vi "CRYHarmonics list to array.vi"(10 "Checkoffs":bool[](array[boolean]), 11 "Harmonic list items":string[](array[string])) -> (2 "List items checked":string[](array[string]), 3 "Harmonics array out":dbl[](array[numeric]) format="%.2f")   [LabVIEW 2013]
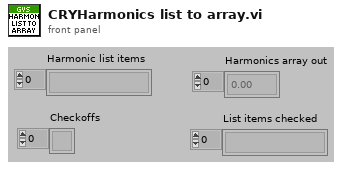
[diagram p1: front panel]
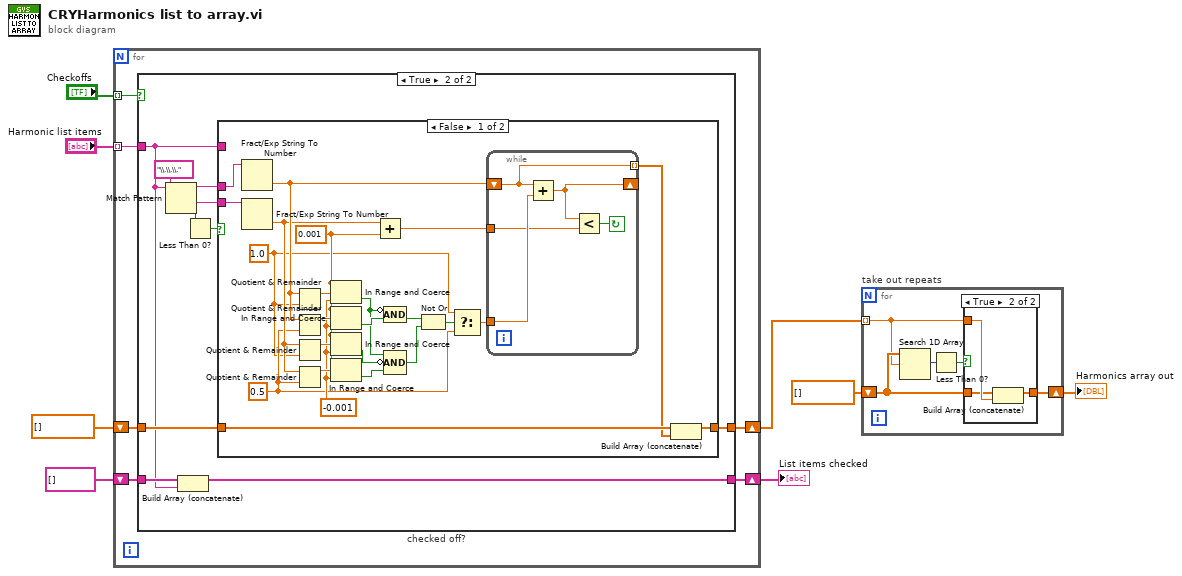
[diagram p0: block diagram]
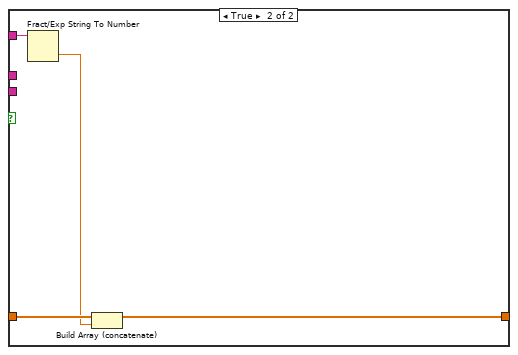
[diagram p4: hidden frame]
diagram:
  n1 = for {
    tunnel: "Checkoffs" -> [w14] mode=indexing
    shift-right: [w11] -> w3
    shift-left: dbl[] [] ("Harmonics array out") -> [w12]
    tunnel: "Harmonic list items" -> [w13] mode=indexing
    shift-right: [w9] -> w4
    shift-left: string[] [] ("Harmonic list items") -> [w10]
    n2 = case "checked off?" shown="True" w14 {
      tunnel: w13 -> [_ w18]
      tunnel: [w16 w20] -> w11
      tunnel: w12 -> [w16 w21]
      tunnel: w10 -> [w15 w19]
      tunnel: [w15 w17] -> w9
      frame False {
      }
      frame True {
        n3 = Match Pattern(string=w18, regular expression="\\.\\.\\.") -> (before substring=w23:string, after substring=w22:string, offset past match=w25:i32)  [unwired: 2 out]
        n4 = Build Array (concatenate)(w19, w18) -> (w17:string[])
        n5 = Less Than 0?(x=w25) -> (x < 0?=w24:bool)
        n6 = case shown="False" w24 {
          tunnel: w23 -> [w50 _]
          tunnel: w22 -> [w49 _]
          tunnel: w21 -> [w42 w59]
          tunnel: w18 -> [_ w58]
          tunnel: [w40 w56] -> w20
          frame False {
            w36 = -0.001
            w37 = 0.001
            w34 = 1.0
            w35 = 0.5
            n7 = Fract/Exp String To Number(string=w50) -> (number=w44:dbl)  [unwired: 4 out]
            n8 = Fract/Exp String To Number(string=w49) -> (number=w39:dbl)  [unwired: 4 out]
            n9 = Quotient & Remainder(x=w44, y=w34) -> (x-y*floor(x/y)=w48:dbl)  [unwired: 1 out]
            n10 = Quotient & Remainder(x=w44, y=w35) -> (x-y*floor(x/y)=w47:dbl)  [unwired: 1 out]
            n11 = Quotient & Remainder(x=w39, y=w34) -> (x-y*floor(x/y)=w38:dbl)  [unwired: 1 out]
            n12 = Quotient & Remainder(x=w39, y=w35) -> (x-y*floor(x/y)=w46:dbl)  [unwired: 1 out]
            n13 = In Range and Coerce(upper limit=w37, x=w48, lower limit=w36) -> (In Range?=w30:bool)  [unwired: 1 out]
            n14 = In Range and Coerce(upper limit=w37, x=w47, lower limit=w36) -> (In Range?=w33:bool)  [unwired: 1 out]
            n15 = In Range and Coerce(upper limit=w37, x=w38, lower limit=w36) -> (In Range?=w31:bool)  [unwired: 1 out]
            n16 = In Range and Coerce(upper limit=w37, x=w46, lower limit=w36) -> (In Range?=w32:bool)  [unwired: 1 out]
            n17 = Add(x=w39, y=w37) -> (x+y=w45:dbl)
            n18 = Compound Arithmetic op=AND(invert w30, w33) -> (w28:bool)
            n19 = Compound Arithmetic op=AND(w30, invert w31, w32) -> (w29:bool)
            n20 = Not Or(1:w29, 2:w28) -> (0:w27:bool)
            n21 = Select(t=w34, s=w27, f=w35) -> (s? t:f=w43:dbl)
            n22 = while {
              tunnel: [w51] -> w41 mode=indexing
              tunnel: w43 -> [w55]
              shift-left: w44 -> [w51]
              shift-right: [w54] -> _
              tunnel: w45 -> [w53]
              stop <- w52 continue-if-true
              n23 = Add(x=w51, y=w55) -> (x+y=w54:dbl)
              n24 = Less?(x=w54, y=w53) -> (x < y?=w52:bool)
            }
            n25 = Build Array (concatenate)(w42, w41) -> (w40:dbl[])
          }
          frame True {
            n26 = Fract/Exp String To Number(string=w58) -> (number=w57:dbl)  [unwired: 4 out]
            n27 = Build Array (concatenate)(w59, w57) -> (w56:dbl[])
          }
        }
      }
    }
  }
  "List items checked" <- w4
  n28 = for "take out repeats" {
    shift-right: [w61] -> w1
    shift-left: dbl[] [] ("Harmonics array out") -> [w62]
    tunnel: w3 -> [w60] mode=indexing
    n29 = Search 1D Array(1D array=w62, element=w60) -> (index of element=w64:i32)  [unwired: 1 out]
    n30 = Less Than 0?(x=w64) -> (x < 0?=w63:bool)
    n31 = case shown="True" w63 {
      tunnel: [w65 w66] -> w61
      tunnel: w62 -> [w65 w67]
      tunnel: w60 -> [_ w68]
      frame False {
      }
      frame True {
        n32 = Build Array (concatenate)(w67, w68) -> (w66:dbl[])
      }
    }
  }
  "Harmonics array out" <- w1
